vi "WFM MNGR Get ET Waveform Name.vi"(8 "error in (no error)":errorcluster, 10 "ET Waveform":T1, 11 "WFM MNGR in":refnum<class "QPA MSMT Waveform Manager.lvclass">) -> (0 "error out":errorcluster, 2 "ET Waveform Name":string, 3 "WFM MNGR out":refnum<class "QPA MSMT Waveform Manager.lvclass">)   [LabVIEW 2016, in "QPA MSMT Waveform Manager.lvclass"]
uses:
  QPA MSMT Waveform Manager.lvclass
  Controls/ET Waveform.ctl
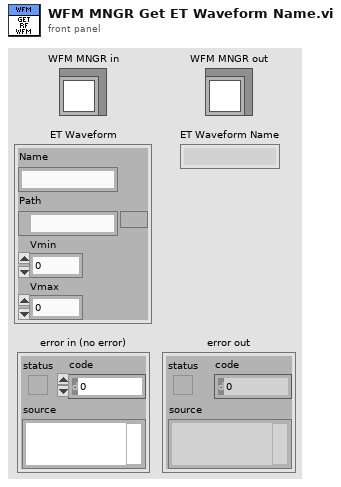
[diagram p1: front panel]
types:
  T1 = typedef "QPA MSMT Waveform Manager.lvclass/ET Waveform.ctl" = cluster{"Name":string, "Path":path, "Vmin":dbl, "Vmax":dbl}
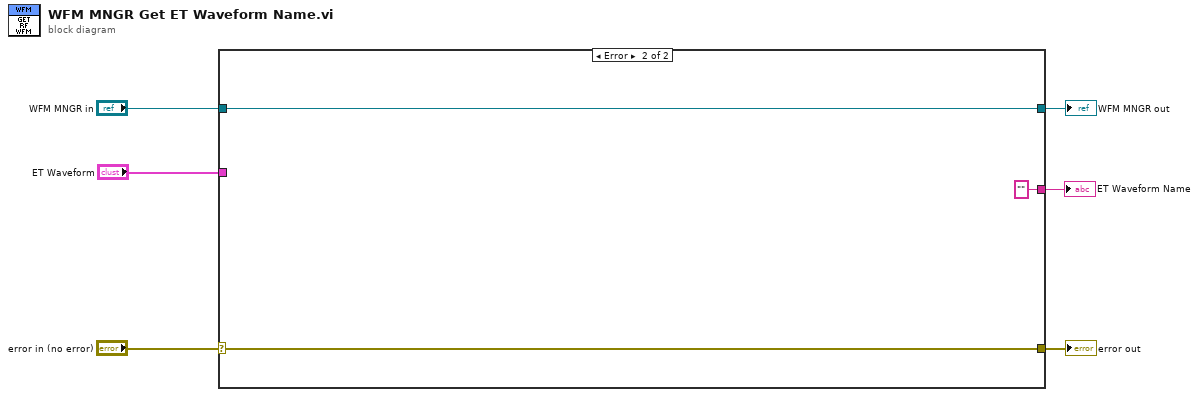
[diagram p0: block diagram]
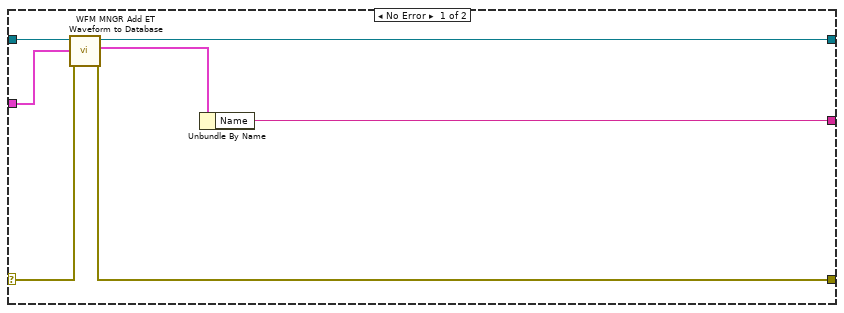
[diagram p2: hidden frame]
diagram:
  n1 = case shown="Error" "error in (no error)" {
    selector: "error in (no error)" -> [w12 w16]
    tunnel: [w11 w16] -> w5
    tunnel: [w10 w15] -> w3
    tunnel: "WFM MNGR in" -> [w13 w15]
    tunnel: "ET Waveform" -> [w8 _]
    tunnel: [w7 "" ("Name")] -> w1
    frame No Error {
      n2 = call "WFM MNGR Add ET Waveform to Database.vi"("error in (no error)"=w12, "ET Waveform"=w8, "WFM MNGR in"=w13) -> ("error out"=w11:errorcluster, "ET Waveform"=w9:T1, "WFM MNGR out"=w10:refnum<class "QPA MSMT Waveform Manager.lvclass">)  [unwired: 6 in]
      n3 = Unbundle By Name(w9) -> ("Name"=w7:string)
    }
    frame Error {
    }
  }
  "error out" <- w5
  "WFM MNGR out" <- w3
  "ET Waveform Name" <- w1
